vi "Duplicate DUT.vi"(8 "error in (no error)":errorcluster, 9 "New DUT Name (\"DUT1-copy\")":string="DUT1-copy", 10 "DUT (\"DUT1\")":string="DUT1", 11 "VISA resource name":refnum<visa-resource-name>) -> (0 "error out":errorcluster, 3 "VISA resource name out":refnum<visa-resource-name>)   [LabVIEW 2020, in "Rohde&Schwarz CMXP Base.lvlib"]
doc: "Creates a DUT with a new name as a copy of the DUT specified.\n\nAttribute:\n-\n\nRemote-control command:\nCOPY:DUT"
uses:
  <instrlib>/Rohde&Schwarz CMXP Base/Rohde&Schwarz CMXP Base.lvlib
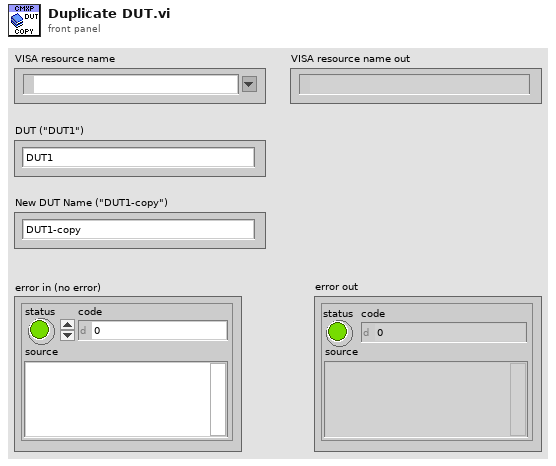
[diagram p1: front panel]
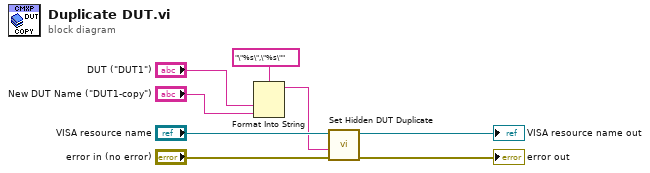
[diagram p0: block diagram]
diagram:
  n1 = Format Into String(format string="\"%s\",\"%s\"", "DUT (\"DUT1\")", "New DUT Name (\"DUT1-copy\")") -> (resulting string=w1:string)  [unwired: 2 in, 1 out]
  n2 = call "Set Hidden DUT Duplicate"("error in (no error)"="error in (no error)", "Hidden DUT Duplicate ()"=w1, "instrument handle"="VISA resource name") -> ("error out"=→"error out":errorcluster, "instrument handle out"=→"VISA resource name out":refnum<visa-resource-name>)  [unwired: 7 in]
